vi "Apply Data To Tree.vi"(6 "Child Position":i32=-1, 8 "error in (no error)":errorcluster, 9 "Tree Item In":T1, 10 "Tree In":refnum<class "Tree.lvclass">, 11 "Composite Tree Data in":refnum<class "Composite Tree Data.lvclass">) -> (0 "error out":errorcluster, 2 "Tree Out":refnum<class "Tree.lvclass">, 3 "Composite Tree Data out":refnum<class "Composite Tree Data.lvclass">)   [LabVIEW 2019, in "Composite Tree Data.lvclass"]
uses:
  Composite Tree Data.lvclass
  Tree/Type Def/Tree Item.ctl
  Tree/Tree.lvclass
  Tree/Tree.lvclass/Tree.ctl
  Composite Tree Data.lvclass/Composite Tree Data.ctl
  Tree/Public Data/Read Root Tag.vi
  Tree Data/Tree Data.lvclass
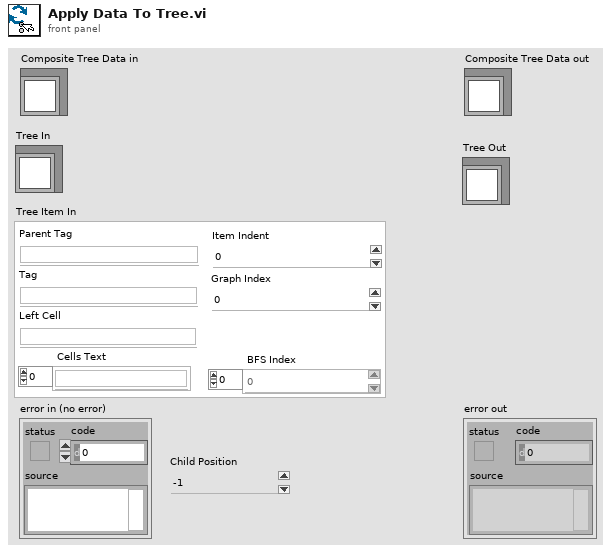
[diagram p1: front panel]
types:
  T1 = typedef "Tree Item.ctl" = cluster{"Parent Tag":string, "Tag":string, "Left Cell":string, "Cells Text":string[], "BFS Index":i32[], "Graph Index":i32, "Item Indent":i32}
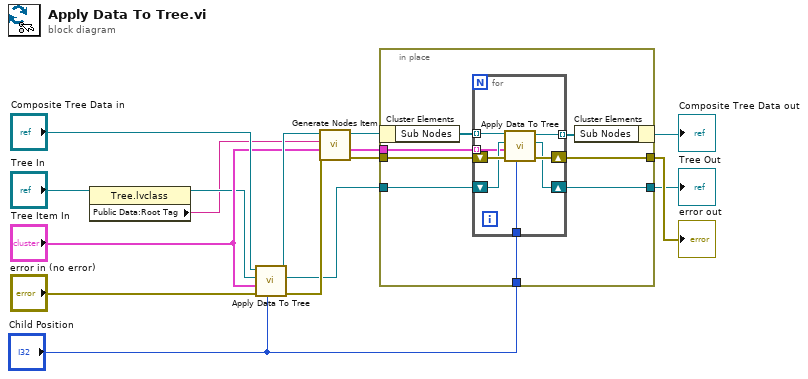
[diagram p0: block diagram]
diagram:
  n1 = property class="Tree.lvclass"(reference="Tree In") -> (reference out=w3:refnum<class "Tree.lvclass">, "Public Data:Root Tag"=w2:string)  [unwired: 1 in, 1 out]
  n2 = call-parent "Apply Data To Tree.vi"("Child Position"="Child Position", "error in (no error)"="error in (no error)", "Tree Item In"="Tree Item In", "Tree In"=w3, "Tree Data in"="Composite Tree Data in") -> ("error out"=w13:errorcluster, "Tree Out"=w9:refnum<class "Tree.lvclass">, "Tree Data out"=w14:refnum<class "Composite Tree Data.lvclass">)  [unwired: 4 in]
  n3 = call-dynamic "Generate Nodes Item.vi"("error in (no error)"=w13, "Tree Item In"="Tree Item In", "Root Tag In"=w2, "Composite Tree Data in"=w14) -> ("error out"=w11:errorcluster, "Nodes Item Out"=w6:T1[], "Composite Tree Data out"=w12:refnum<class "Composite Tree Data.lvclass">)  [unwired: 5 in]
  n4 = in-place {
    in-place-border: w11 -> [w22]
    in-place-border: w9 -> [w21]
    in-place-border: [w20] -> w8
    in-place-border: [w19] -> w7
    in-place-border: w6 -> [w18]
    in-place-border: "Child Position" -> [w17]
    n5 = in-place-cluster #1(w12) -> ("Sub Nodes"=w24:refnum<class "Tree Data.lvclass">[])
    n6 = for {
      tunnel: w24 -> [w32] mode=indexing
      tunnel: [w31] -> w23 mode=indexing
      shift-right: [w29] -> w20
      shift-left: w22 -> [w30]
      shift-right: [w27] -> w19
      shift-left: w21 -> [w28]
      tunnel: w18 -> [w26] mode=indexing
      tunnel: w17 -> [w25]
      n7 = call-dynamic "Apply Data To Tree.vi"("Child Position"=w25, "error in (no error)"=w30, "Tree Item In"=w26, "Tree In"=w28, "Tree Data in"=w32) -> ("error out"=w29:errorcluster, "Tree Out"=w27:refnum<class "Tree.lvclass">, "Tree Data out"=w31:refnum<class "Tree Data.lvclass">)  [unwired: 4 in]
    }
    n8 = in-place-cluster #1("Sub Nodes"=w23) -> (→"Composite Tree Data out":refnum<class "Composite Tree Data.lvclass">)
  }
  "error out" <- w8
  "Tree Out" <- w7
